vi "Initialize.vi"(8 "error in":errorcluster, 10 "parameters":variant, 11 "node in":refnum<class "TBM Configuration Node.lvclass">) -> (0 "error out":errorcluster, 2 "summary":T2[](array[typedef]), 3 "data value reference":T1)   [LabVIEW 2013, in "PL Framework Configuration Tool.lvlib" / "TBM Configuration Node.lvclass"]
doc: "Initializes the data of a node to its default state.\nThe object is not created inside of this VI, because it is created from a File depending on user selection."
uses:
  TBM Configuration Node.lvclass
  <vilib>/CEF_TreeControl/Node/Summary.ctl
  <vilib>/CEF_TreeControl/Node/NodeRef.ctl
  <vilib>/CEF_TreeControl/Node/NISE_CEF_Node.lvclass
  <vilib>/NI/Tag Bus Module Framework/root configuration/TBM configuration.lvclass
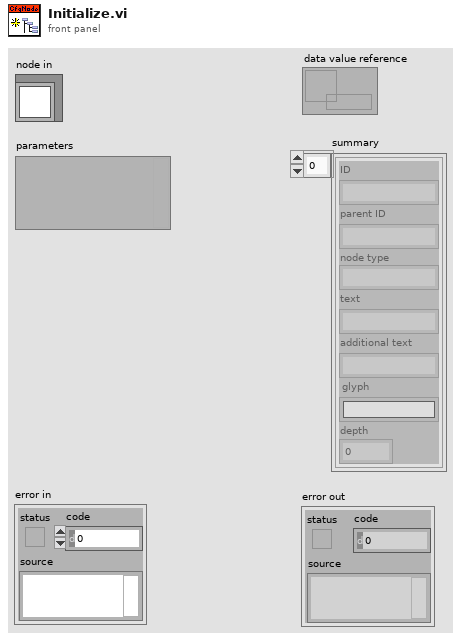
[diagram p1: front panel]
types:
  T1 = typedef "NISE_CEF_Node.lvclass/NodeRef.ctl" = refnum<data-value>
  T2 = typedef "NISE_CEF_Node.lvclass/Summary.ctl" = cluster{"ID":string, "parent ID":string, "node type":string, "text":string, "additional text":string, "glyph":string, "depth":i32}
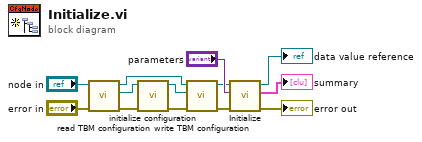
[diagram p0: block diagram]
diagram:
  n1 = call-dynamic "read TBM configuration.vi"("error in"="error in", "TBM Configuration Node in"="node in") -> ("error out"=w6:errorcluster, "configuration"=w9:refnum<class "TBM configuration.lvclass">, "TBM Configuration Node out"=w7:refnum<class "TBM Configuration Node.lvclass">)  [unwired: 7 in]
  n2 = call-dynamic "initialize configuration.vi"("error in"=w6, "configuration in"=w9) -> ("error out"=w5:errorcluster, "configuration out"=w8:refnum<class "TBM configuration.lvclass">)  [unwired: 7 in, 1 out]
  n3 = call-dynamic "write TBM configuration.vi"("error in"=w5, "configuration"=w8, "TBM Configuration Node in"=w7) -> ("error out"=w4:errorcluster, "TBM Configuration Node out"=w3:refnum<class "TBM Configuration Node.lvclass">)  [unwired: 7 in]
  n4 = call-parent "Initialize.vi"("error in"=w4, "parameters"="parameters", "node in"=w3) -> ("error out"=→"error out":errorcluster, "summary"=→"summary":T2[], "data value reference"=→"data value reference":T1)  [unwired: 6 in]
